vi "ButtonRemoveTotes.vi"(11 "array":dbl[](array[numeric])) -> ()   [LabVIEW 2014]
uses:
  Gantry/GantryGlobals.vi
  ToteCount.vi
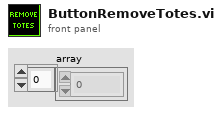
[diagram p1: front panel]
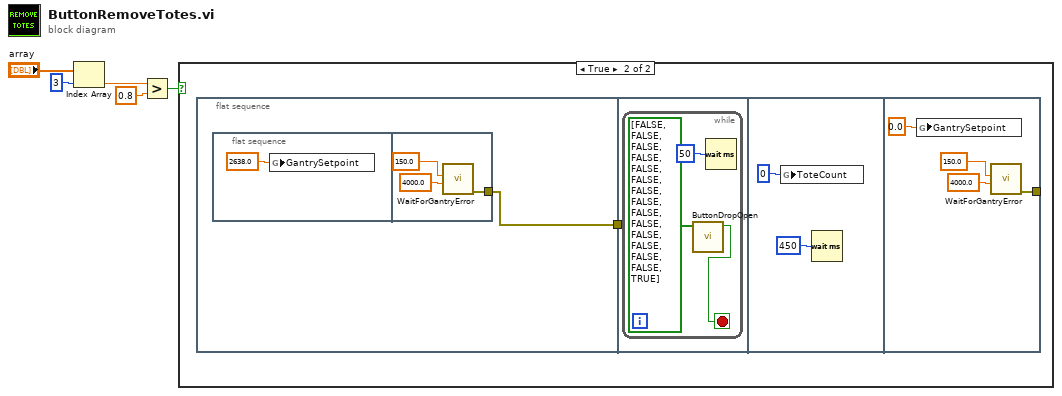
[diagram p0: block diagram]
diagram:
  n1 = Index Array(array="array", index=3) -> (element=w3:dbl)
  n2 = Greater?(x=w3, y=0.8) -> (0:w1:bool)
  n3 = case shown="True" w1 {
    frame False {
    }
    frame True {
      n4 = flat-sequence {
        tunnel: [w7] -> w6
        tunnel: w6 -> [_]
        tunnel: [w17] -> _
        frame #0 {
          n5 = flat-sequence {
            tunnel: [w9] -> w7
            frame #0 {
              n6 = global write "GantryGlobals.vi" "GantrySetpoint"(2638.0 ("GantrySetpoint")) -> ()
            }
            frame #1 {
              n7 = call "WaitForGantryError.vi"("Timeout (ms)"=4000.0, "AllowedError"=150.0) -> ("error out"=w9:errorcluster)  [unwired: 9 in]
            }
          }
        }
        frame #1 {
          n8 = while {
            stop <- w13 stop-if-true
            n9 = call "ButtonDropOpen.vi"("Buttons"=bool[] [FALSE, FALSE, FALSE, FALSE, FALSE, FALSE, FALSE, FALSE, FALSE, FALSE, FALSE, FALSE, FALSE, FALSE, TRUE]) -> ("Boolean"=w13:bool)  [unwired: 10 in]
            n10 = Wait (ms)(milliseconds to wait=u32 50) -> ()  [unwired: 1 out]
          }
        }
        frame #2 {
          n11 = global write "ToteCount.vi" "ToteCount"(0 ("ToteCount")) -> ()
          n12 = Wait (ms)(milliseconds to wait=u32 450) -> ()  [unwired: 1 out]
        }
        frame #3 {
          n13 = global write "GantryGlobals.vi" "GantrySetpoint"(0.0 ("GantrySetpoint")) -> ()
          n14 = call "WaitForGantryError.vi"("Timeout (ms)"=4000.0, "AllowedError"=150.0) -> ("error out"=w17:errorcluster)  [unwired: 9 in]
        }
      }
    }
  }
